vi "setRangeXml.vi"(8 "error in (no error)":errorcluster, 10 "rangeInUse_xmlNode":refnum<class "xmlNode.lvclass">, 11 "AnalogDevice in":refnum<class "AnalogDevice.lvclass">) -> (0 "error out":errorcluster, 3 "AnalogDevice out":refnum<class "AnalogDevice.lvclass">)   [LabVIEW 2009, in "Tools.lvlib" / "DatabaseHelpers.lvlib" / "AnalogDevice.lvclass"]
uses:
  AnalogDevice.lvclass
  xmlNode/xmlNode.lvclass
  AnalogDevice.lvclass/AnalogDevice.ctl
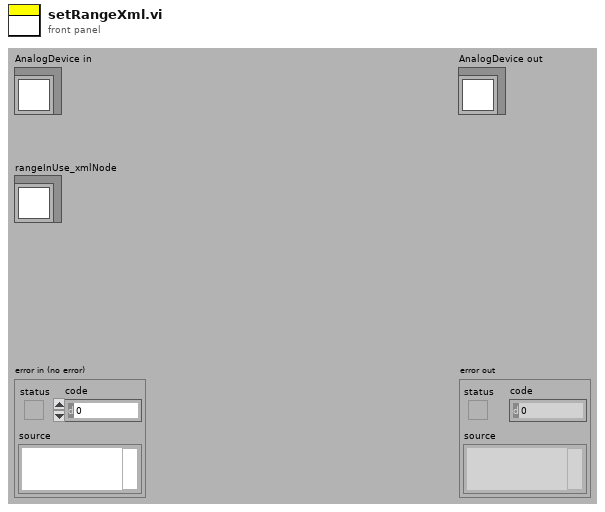
[diagram p1: front panel]
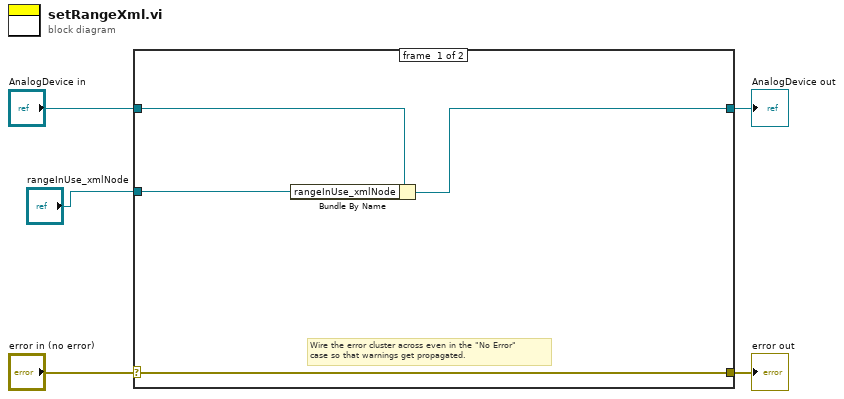
[diagram p0: block diagram]
diagram:
  n1 = case shown="No Error" "error in (no error)" {
    selector: "error in (no error)" -> [w9 w11]
    tunnel: [w9 w11] -> w4
    tunnel: [w7 w10] -> w2
    tunnel: "AnalogDevice in" -> [w8 w10]
    tunnel: "rangeInUse_xmlNode" -> [w6 _]
    frame #0 {
      # "Wire the error cluster across even in the \"No Error\"\ncase so that warnings get propagated."
      n2 = Bundle By Name(cluster=w8, "rangeInUse_xmlNode"=w6) -> (w7:refnum<class "AnalogDevice.lvclass">)
    }
    frame #1 {
    }
  }
  "error out" <- w4
  "AnalogDevice out" <- w2
